vi "Read CFG File.vi"(7 "Section":string, 8 "error in (no error)":errorcluster, 10 "File refnum":T1, 11 "Mag Lab Parameters in":refnum<class "Mag Lab Parameters.lvclass">) -> (0 "error out":errorcluster, 2 "File refnum out":T1, 3 "Mag Lab Parameters out":refnum<class "Mag Lab Parameters.lvclass">)   [LabVIEW 2015, in "Mag Lab Parameters.lvclass"]
uses:
  Mag Lab Parameters.lvclass
  <vilib>/Utility/config.llb/Config Data RefNum.ctl
  <vilib>/Utility/config.llb/NI_LVConfig.lvlib
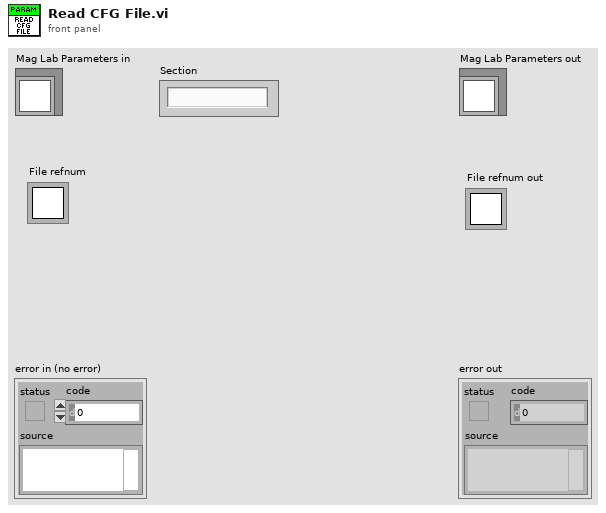
[diagram p1: front panel]
types:
  T1 = typedef "NI_LVConfig.lvlib/Config Data RefNum.ctl" = refnum<k1>
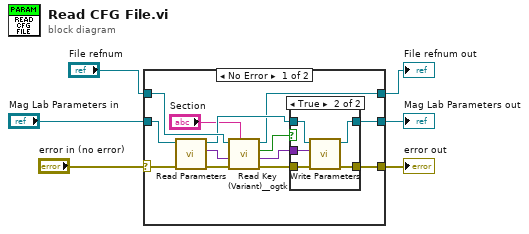
[diagram p0: block diagram]
diagram:
  n1 = case shown="No Error" "error in (no error)" {
    selector: "error in (no error)" -> [w8 w29]
    tunnel: [w9 w29] -> w5
    tunnel: [w13 w28] -> w3
    tunnel: "Mag Lab Parameters in" -> [w19 w28]
    tunnel: "File refnum" -> [w18 w27]
    tunnel: [w14 w27] -> w1
    frame No Error {
      n2 = call-dynamic "Read Parameters.vi"("error in (no error)"=w8, "Mag Lab Parameters in"=w19) -> ("error out"=w7:errorcluster, "Parameters"=w16:variant, "Mag Lab Parameters out"=w17:refnum<class "Mag Lab Parameters.lvclass">)  [unwired: 7 in]
      n3 = call <userlib>:"Read Key (Variant)__ogtk.vi"("section"="Section", "error in (no error)"=w7, "type"=w16, "refnum"=w18) -> ("error out"=w10:errorcluster, "key-value"=w12:variant, "found?"=w11:bool, "refnum out"=w14:T1)  [unwired: 4 in]
      n4 = case shown="True" w11 {
        tunnel: w17 -> [w21 w26]
        tunnel: [w21 w25] -> w13
        tunnel: w12 -> [_ w24]
        tunnel: w10 -> [w20 w23]
        tunnel: [w20 w22] -> w9
        frame False {
        }
        frame True {
          n5 = call-dynamic "Write Parameters.vi"("error in (no error)"=w23, "Parameters"=w24, "Mag Lab Parameters in"=w26) -> ("error out"=w22:errorcluster, "Mag Lab Parameters out"=w25:refnum<class "Mag Lab Parameters.lvclass">)  [unwired: 7 in]
        }
      }
    }
    frame Error {
    }
  }
  "error out" <- w5
  "Mag Lab Parameters out" <- w3
  "File refnum out" <- w1
